vi "Drive_arc.vi"() -> ()   [LabVIEW 2017, in "labview-standard-library.lvlib" / "automode-scripting.lvlib"]
uses:
  automode-scripting.lvlib
panel:
  in  "0=left 1=right":u8
  in  "0=reverse 1=forward":u8
  in  "Wheel base":dbl
  out "Left side out":dbl
  out "Right side out":dbl
  in  "Radius":dbl
  in  "Angle":dbl
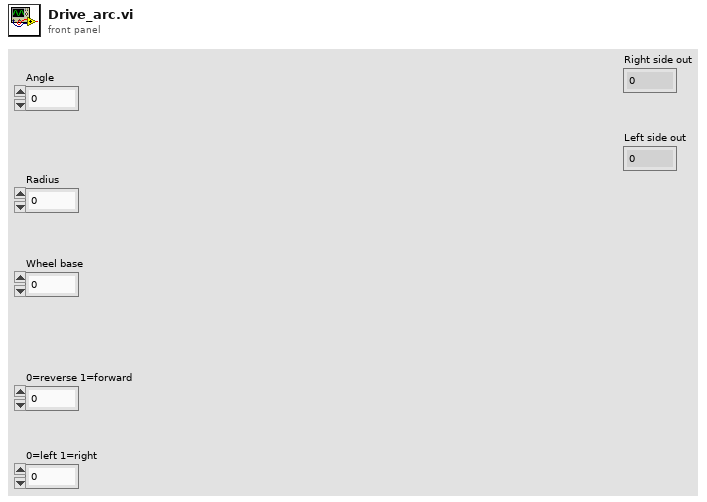
[diagram p1: front panel]
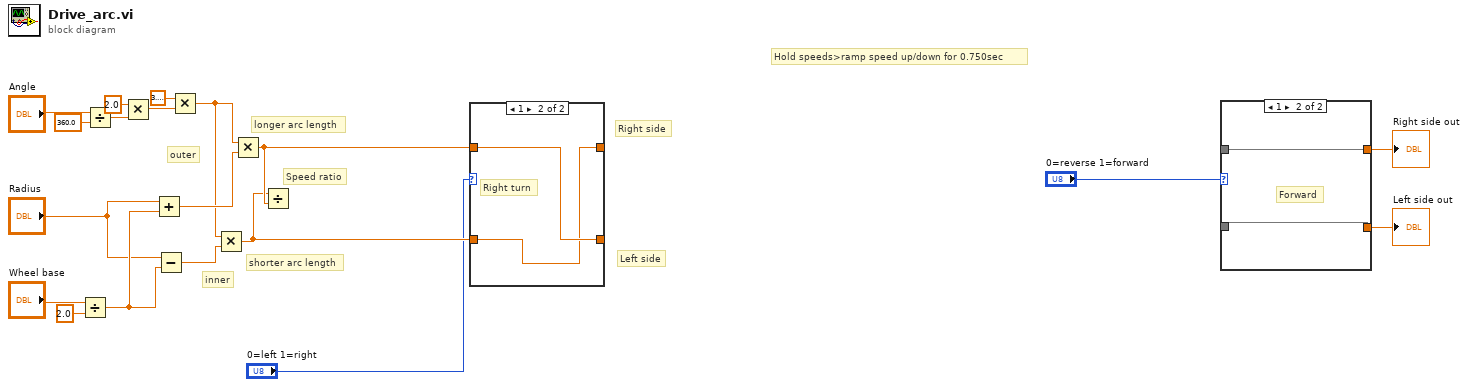
[diagram p0: block diagram]
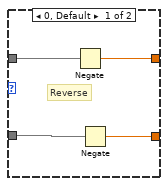
[diagram p2: hidden frame]
diagram:
  # "Hold speeds>ramp speed up/down for 0.750sec"
  # "Left side"
  # "Right side"
  # "shorter arc length"
  # "longer arc length"
  # "Speed ratio"
  # "inner"
  # "outer"
  n1 = Divide(x="Wheel base", y=2.0) -> (x/y=w11:dbl)
  n2 = Divide(x="Angle", y=360.0) -> (x/y=w17:dbl)
  n3 = Multiply(x=2.0, y=w17) -> (x*y=w15:dbl)
  n4 = Add(x="Radius", y=w11) -> (x+y=w9:dbl)
  n5 = Subtract(x="Radius", y=w11) -> (x-y=w8:dbl)
  n6 = Multiply(x=3.141592653589793, y=w15) -> (x*y=w7:dbl)
  n7 = Multiply(x=w7, y=w8) -> (x*y=w5:dbl)
  n8 = Multiply(x=w7, y=w9) -> (x*y=w6:dbl)
  n9 = Divide(x=w5, y=w6) -> ()  [unwired: 1 out]
  n10 = case shown="1" "0=left 1=right" {
    tunnel: w6 -> [w21 w23]
    tunnel: w5 -> [w20 w22]
    tunnel: [w21 w22] -> _
    tunnel: [w20 w23] -> _
    frame 0, Default {
      # "Left turn"
    }
    frame 1 {
      # "Right turn"
    }
  }
  n11 = case shown="1" "0=reverse 1=forward" {
    tunnel: [w27 w29] -> w3
    tunnel: [w26 w28] -> w2
    tunnel: _ -> [w25 w29]
    tunnel: _ -> [w24 w28]
    frame 0, Default {
      # "Reverse"
      n12 = Negate(x=w25) -> (-x=w27:dbl)
      n13 = Negate(x=w24) -> (-x=w26:dbl)
    }
    frame 1 {
      # "Forward"
    }
  }
  "Right side out" <- w3
  "Left side out" <- w2
